vi "Day 3.vi"() -> ()   [LabVIEW 2020]
panel:
  in  "Path":path=path "D:/gitRepo/AdventofCode-2020-LabVIEW/Inputs/Day 3.txt"
  out "product":u32
  out "Trees Per Route":u32[](array[numeric])
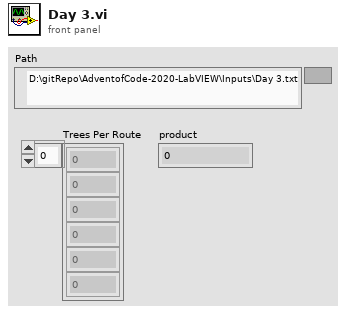
[diagram p1: front panel]
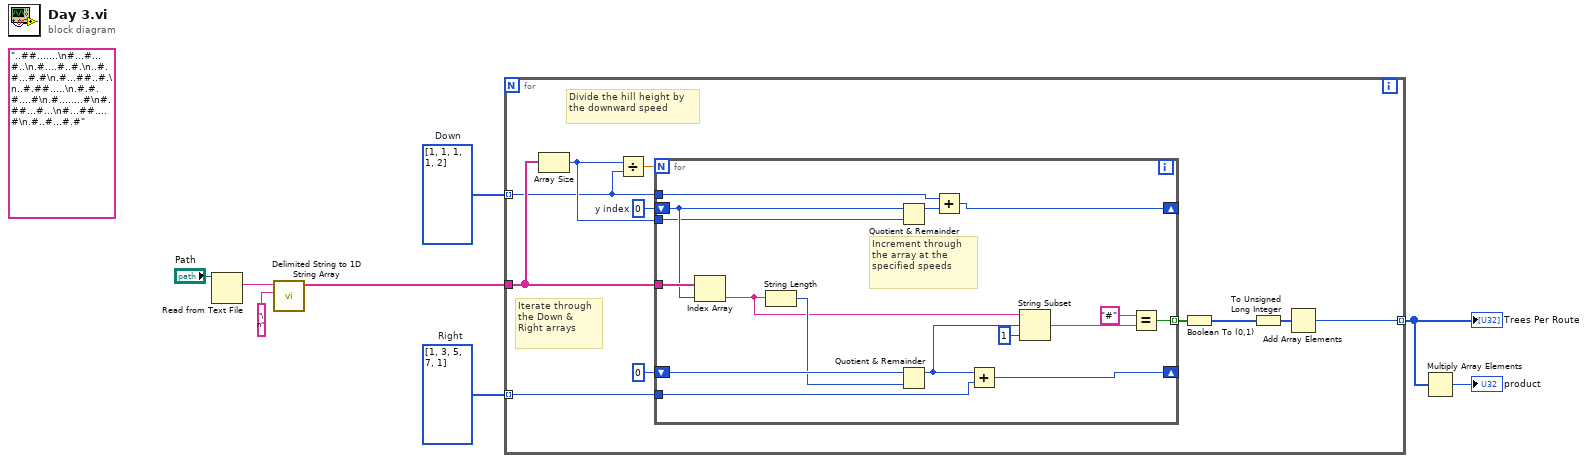
[diagram p0: block diagram]
diagram:
  w7 = i32[] [1, 1, 1, 1, 2]  # Down
  w6 = i32[] [1, 3, 5, 7, 1]  # Right
  (unwired) "..##.......\n#...#...#..\n.#....#..#.\n..#.#...#.#\n.#...##..#.\n..#.##.....\n.#.#.#....#\n.#........#\n#.##...#...\n#...##....#\n.#..#...#.#"
  n1 = Read from Text File(file (use dialog)="Path") -> (text=w3:string)  [unwired: 3 in, 3 out]
  n2 = call <vilib>:"Delimited String to 1D String Array.vi"("delimiter"="\n" ("delimiter (Tab)"), "delimited string"=w3) -> ("string array"=w1:string[])  [unwired: 9 in]
  n3 = for {
    tunnel: w1 -> [w17]
    tunnel: [w14] -> w5 mode=indexing
    tunnel: w7 -> [w9] mode=indexing
    tunnel: w6 -> [w13] mode=indexing
    w18 = 0  # y index
    # "Divide the hill height by the downward speed"
    # "Iterate through the Down & Right arrays"
    n4 = Array Size(array=w17) -> (size(s)=w11:i32)
    n5 = Divide(x=w11, y=w9) -> (x/y=w10:dbl)
    n6 = for {
      N: w10 -> [_]
      shift-right: [w31] -> _
      shift-left: 0 -> [w35]
      shift-right: [w21] -> _
      shift-left: w18 -> [w23]
      tunnel: w17 -> [w24]
      tunnel: w11 -> [w20]
      tunnel: [w27] -> w16 mode=indexing
      tunnel: w9 -> [w26]
      tunnel: w13 -> [w25]
      # "Increment through the array at the specified speeds"
      n7 = Index Array "Index Array"(array=w24, index=w23) -> (element=w22:string)
      n8 = String Length(string=w22) -> (length=w33:i32)
      n9 = Quotient & Remainder(x=w23, y=w20) -> (x-y*floor(x/y)=w34:i32)  [unwired: 1 out]
      n10 = Quotient & Remainder(x=w35, y=w33) -> (x-y*floor(x/y)=w30:i32)  [unwired: 1 out]
      n11 = Add(x=w26, y=w34) -> (x+y=w21:i32)
      n12 = Add(x=w30, y=w25) -> (x+y=w31:i32)
      n13 = String Subset(string=w22, offset (0)=w30, length (rest)=1 ("length (rest)")) -> (substring=w29:string)
      n14 = Equal?(x="#", y=w29) -> (x = y?=w27:bool)
    }
    n15 = Boolean To (0,1)(Boolean=w16) -> (0, 1=w15:i16[])
    n16 = To Unsigned Long Integer(number=w15) -> (unsigned 32bit integer=w12:u32[])
    n17 = Add Array Elements(numeric array=w12) -> (sum=w14:u32)
  }
  "Trees Per Route" <- w5
  n18 = Multiply Array Elements(1:w5) -> (0:→"product":u32)
